vi "Choose Build Spec.vi"(8 "error in":errorcluster, 10 "Build Type":T2, 11 "Build Specs":T1[](array[typedef])=[{"Name"="My Application", "Type"="EXE", "Version"="1.0.0.1"}, {"Name"="My Installer", "Type"="Installer", "Version"="1.0.0"}, {"Name"="My Interop Assembly", "Type"=".NET Interop Assembly", "Version"="1"}, {"Name"="My Package", "Type"="{E661DAE2-7517-431F-AC41-30807A3BDA38}", "Version"="0"}, {"Name"="My Packed Library", "Type"="Packed Library", "Version"="1"}, {"Name"="My DLL", "Type"="DLL", "Version"="1"}, {"Name"="My Source Distribution", "Type"="Source Distribution", "Version"="1"}, {"Name"="My Zip File", "Type"="Zip File", "Version"="0"}]) -> (0 "error out":errorcluster, 1 "Version":string, 2 "Name":string, 3 "Build Specs out":T1[](array[typedef])=[{"Name"="My Application", "Type"="EXE", "Version"="1.0.0.1"}, {"Name"="My Installer", "Type"="Installer", "Version"="1.0.0"}, {"Name"="My Interop Assembly", "Type"=".NET Interop Assembly", "Version"="1"}, {"Name"="My Package", "Type"="{E661DAE2-7517-431F-AC41-30807A3BDA38}", "Version"="0"}, {"Name"="My Packed Library", "Type"="Packed Library", "Version"="1"}, {"Name"="My DLL", "Type"="DLL", "Version"="1"}, {"Name"="My Source Distribution", "Type"="Source Distribution", "Version"="1"}, {"Name"="My Zip File", "Type"="Zip File", "Version"="0"}])   [LabVIEW 2019, in "Build.lvlib"]
uses:
  Build.lvlib
  Typedefs/Build Spec Type--combo.ctl
  Typedefs/Build Spec--cluster.ctl
  <vilib>/Utility/error.llb/Error Cluster From Error Code.vi
  <vilib>/ErrorRing/Error Ring.xnode
panel:
  out "Type":string
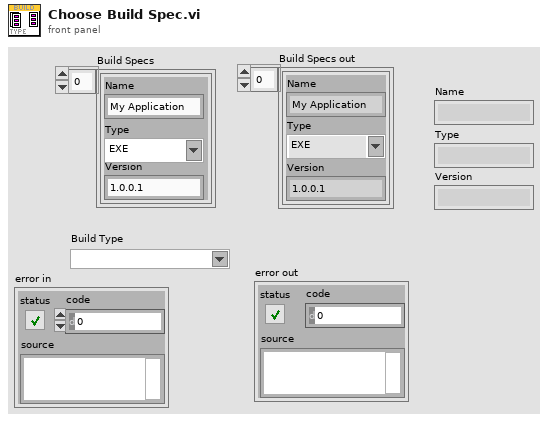
[diagram p1: front panel]
types:
  T1 = typedef "Build.lvlib/Build Spec--cluster.ctl" = cluster{"Name":string, "Type":string, "Version":string}
  T2 = typedef "Build.lvlib/Build Spec Type--combo.ctl" = string
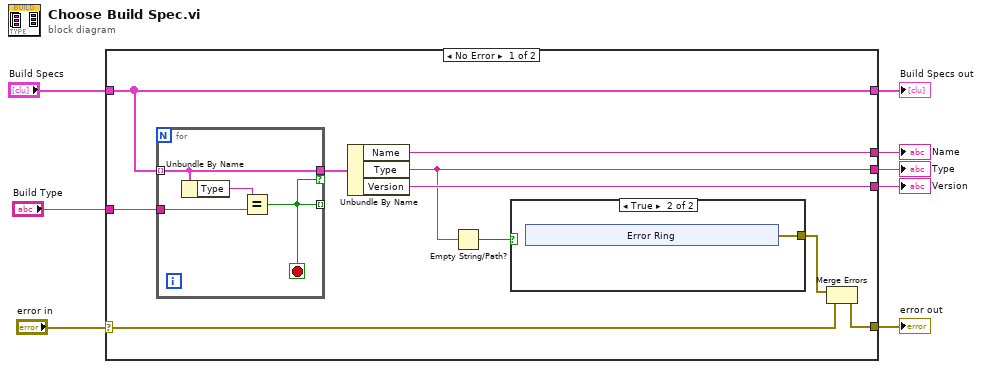
[diagram p0: block diagram]
diagram:
  n1 = case shown="No Error" "error in" {
    selector: "error in" -> [w13 w28]
    tunnel: "Build Type" -> [w18 _]
    tunnel: [w16 _] -> w7
    tunnel: [w15 _] -> w6
    tunnel: "Build Specs" -> [w9 w29]
    tunnel: [w12 _] -> w3
    tunnel: [w10 w28] -> w2
    tunnel: [w9 w29] -> w1
    frame No Error {
      n2 = for {
        tunnel: w18 -> [w26]
        tunnel: w9 -> [w25] mode=indexing
        tunnel: [w24] -> _ mode=indexing
        tunnel: [w25] -> w17 if=w24
        stop <- w24 stop-if-true
        n3 = Unbundle By Name(w25) -> ("Type"=w27:string)
        n4 = Equal?(x=w27, y=w26) -> (x = y?=w24:bool)
      }
      n5 = Unbundle By Name(w17) -> ("Name"=w16:string, "Type"=w12:string, "Version"=w15:string)
      n6 = Empty String/Path?(string/path=w12) -> (empty?=w14:bool)
      n7 = case shown="True" w14 {
        tunnel: [_ w19] -> w11
        frame False {
        }
        frame True {
          n8 = xnode "Error Ring"() -> ("error out"=w19:errorcluster)
        }
      }
      n9 = Merge Errors(w11, w13) -> (w10:errorcluster)
    }
    frame Error {
    }
  }
  "Build Specs out" <- w1
  "Name" <- w7
  "Type" <- w3
  "Version" <- w6
  "error out" <- w2
